vi "Valve Channel.vi"(8 "error in (no error)":errorcluster) -> (0 "error out":errorcluster, 3 "Refnum out":refnum<k21>)   [LabVIEW 2019]
uses:
  <vilib>/DAQmx/create/channels.llb/DAQmx Create Channel (DO-Digital Output).vi
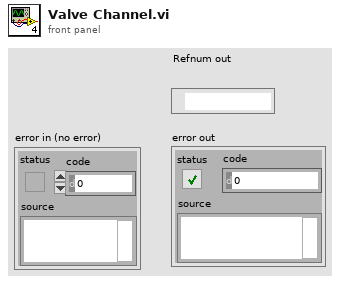
[diagram p1: front panel]
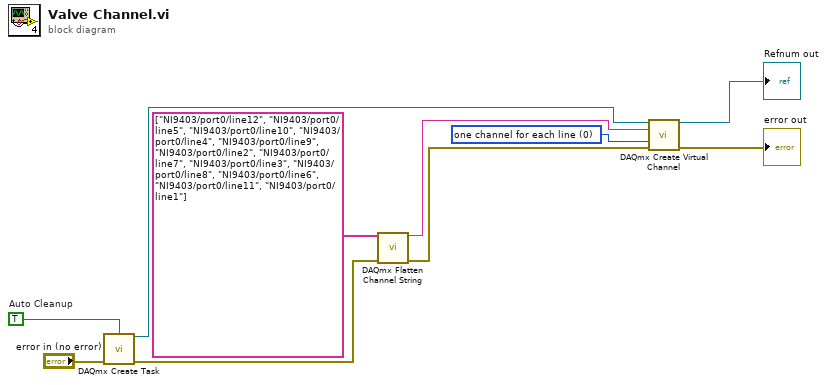
[diagram p0: block diagram]
diagram:
  w6 = 0 items=["one channel for each line", "one channel for all lines"] ("line grouping")
  w5 = TRUE  # Auto Cleanup
  n1 = call <vilib>:"DAQmx Create Task.vi"("auto cleanup"=w5, "error in"="error in (no error)") -> ("task out"=w4:refnum<k21>, "error out"=w9:errorcluster)  [unwired: 12 in]
  n2 = call <vilib>:"DAQmx Flatten Channel String.vi"("names in"=tag[] ["NI9403/port0/line12", "NI9403/port0/line5", "NI9403/port0/line10", "NI9403/port0/line4", "NI9403/port0/line9", "NI9403/port0/line2", "NI9403/port0/line7", "NI9403/port0/line3", "NI9403/port0/line8", "NI9403/port0/line6", "NI9403/port0/line11", "NI9403/port0/line1"] ("lines"), "error in"=w9) -> ("names out"=w8:string, "error out"=w10:errorcluster)  [unwired: 12 in]
  n3 = call-poly <vilib>:"DAQmx Create Virtual Channel.vi"("task in"=w4, "lines"=w8, "line grouping"=w6, "error in"=w10) -> ("task out"=→"Refnum out":refnum<k21>, "error out"=→"error out":errorcluster)  [unwired: 10 in]
